vi "Main.vi"() -> ()   [LabVIEW 2021] (continued)
                    n1024 = String Subset(string=w1278, length (rest)=16 ("长度（剩余）")) -> (substring=w1277:string)  [unwired: 1 in]
                    n1025 = property on="曲线49设置" class="Str"("Val(Sgnl)"=w1277) -> ()  [unwired: 2 in, 2 out]
                    n1026 = invoke on="控件配置文件" class="Tbl (严格)" method="Set Cell Value"("X Index"=1 ("X索引"), "Y Index"=w1272, "Value"=w1279) -> ()  [unwired: 3 in, 6 out]
                    n1027 = invoke on="控件配置文件" class="Tbl (严格)" method="Set Cell Value"("X Index"=0 ("X索引"), "Y Index"=w1272, "Value"=w1277) -> ()  [unwired: 3 in, 6 out]
                  }
                  frame "关联到曲线50" {
                    w1283 = T9 79 items=["刷新间隔", "波特率", "布尔1设置项", "布尔2设置项", "布尔3设置项", "布尔4设置项", "布尔5设置项", "布尔6设置项", "布尔7设置项", "布尔8设置项", "显控1设置", "显控2设置", "显控3设置", "显控4设置", "显控5设置", "显控6设置", "显控7设置", "显控8设置", "显控9设置", "显控10设置", "显控11设置", "显控12设置", "设控1设置", "设控2设置", "设控3设置", "设控4设置", "设控5设置", "设控6设置", "设控7设置", "设控8设置", "曲线1设置", "曲线2设置", "曲线3设置", "曲线4设置", "曲线5设置", "曲线6设置", "曲线7设置", "曲线8设置", "曲线9设置", "曲线10设置", "曲线11设置", "曲线12设置", "曲线13设置", "曲线14设置", "曲线15设置", "曲线16设置", "曲线17设置", "曲线18设置", "曲线19设置", "曲线20设置", "曲线21设置", "曲线22设置", "曲线23设置", "曲线24设置", "曲线25设置", "曲线26设置", "曲线27设置", "曲线28设置", "曲线29设置", "曲线30设置", "曲线31设置", "曲线32设置", "曲线33设置", "曲线34设置", "曲线35设置", "曲线36设置", "曲线37设置", "曲线38设置", "曲线39设置", "曲线40设置", "曲线41设置", "曲线42设置", "曲线43设置", "曲线44设置", "曲线45设置", "曲线46设置", "曲线47设置", "曲线48设置", "曲线49设置", "曲线50设置", "曲线51设置", "曲线52设置", "曲线53设置", "曲线54设置", "曲线55设置", "曲线56设置", "曲线57设置", "曲线58设置", "曲线59设置", "曲线60设置", "曲线61设置", "曲线62设置", "曲线63设置", "曲线64设置", "ID值", "数据模式"] ("DataInitDef")
                    n1028 = property on="表格" class="Tbl (严格)"() -> ("Selection Start"=w1293:T1)  [unwired: 2 in, 2 out]
                    n1029 = Unbundle By Name(w1293) -> ("Row"=w1291:i32)
                    n1030 = property on="表格" class="Tbl (严格)"() -> ("Value"=w1292:string[][])  [unwired: 2 in, 2 out]
                    n1031 = Number To Decimal String(number=w1291) -> (decimal integer string=w1290:string)  [unwired: 1 in]
                    n1032 = Index Array(array=w1292, index (row)=w1291, index (col)=0 ("禁用的索引 (列)")) -> (element=w1289:string)
                    n1033 = String Subset(string=w1289, length (rest)=16 ("长度（剩余）")) -> (substring=w1288:string)  [unwired: 1 in]
                    n1034 = property on="曲线50设置" class="Str"("Val(Sgnl)"=w1288) -> ()  [unwired: 2 in, 2 out]
                    n1035 = invoke on="控件配置文件" class="Tbl (严格)" method="Set Cell Value"("X Index"=1 ("X索引"), "Y Index"=w1283, "Value"=w1290) -> ()  [unwired: 3 in, 6 out]
                    n1036 = invoke on="控件配置文件" class="Tbl (严格)" method="Set Cell Value"("X Index"=0 ("X索引"), "Y Index"=w1283, "Value"=w1288) -> ()  [unwired: 3 in, 6 out]
                  }
                  frame "关联到曲线51" {
                    w1294 = T9 80 items=["刷新间隔", "波特率", "布尔1设置项", "布尔2设置项", "布尔3设置项", "布尔4设置项", "布尔5设置项", "布尔6设置项", "布尔7设置项", "布尔8设置项", "显控1设置", "显控2设置", "显控3设置", "显控4设置", "显控5设置", "显控6设置", "显控7设置", "显控8设置", "显控9设置", "显控10设置", "显控11设置", "显控12设置", "设控1设置", "设控2设置", "设控3设置", "设控4设置", "设控5设置", "设控6设置", "设控7设置", "设控8设置", "曲线1设置", "曲线2设置", "曲线3设置", "曲线4设置", "曲线5设置", "曲线6设置", "曲线7设置", "曲线8设置", "曲线9设置", "曲线10设置", "曲线11设置", "曲线12设置", "曲线13设置", "曲线14设置", "曲线15设置", "曲线16设置", "曲线17设置", "曲线18设置", "曲线19设置", "曲线20设置", "曲线21设置", "曲线22设置", "曲线23设置", "曲线24设置", "曲线25设置", "曲线26设置", "曲线27设置", "曲线28设置", "曲线29设置", "曲线30设置", "曲线31设置", "曲线32设置", "曲线33设置", "曲线34设置", "曲线35设置", "曲线36设置", "曲线37设置", "曲线38设置", "曲线39设置", "曲线40设置", "曲线41设置", "曲线42设置", "曲线43设置", "曲线44设置", "曲线45设置", "曲线46设置", "曲线47设置", "曲线48设置", "曲线49设置", "曲线50设置", "曲线51设置", "曲线52设置", "曲线53设置", "曲线54设置", "曲线55设置", "曲线56设置", "曲线57设置", "曲线58设置", "曲线59设置", "曲线60设置", "曲线61设置", "曲线62设置", "曲线63设置", "曲线64设置", "ID值", "数据模式"] ("DataInitDef")
                    n1037 = property on="表格" class="Tbl (严格)"() -> ("Selection Start"=w1304:T1)  [unwired: 2 in, 2 out]
                    n1038 = Unbundle By Name(w1304) -> ("Row"=w1302:i32)
                    n1039 = property on="表格" class="Tbl (严格)"() -> ("Value"=w1303:string[][])  [unwired: 2 in, 2 out]
                    n1040 = Number To Decimal String(number=w1302) -> (decimal integer string=w1301:string)  [unwired: 1 in]
                    n1041 = Index Array(array=w1303, index (row)=w1302, index (col)=0 ("禁用的索引 (列)")) -> (element=w1300:string)
                    n1042 = String Subset(string=w1300, length (rest)=16 ("长度（剩余）")) -> (substring=w1299:string)  [unwired: 1 in]
                    n1043 = property on="曲线51设置" class="Str"("Val(Sgnl)"=w1299) -> ()  [unwired: 2 in, 2 out]
                    n1044 = invoke on="控件配置文件" class="Tbl (严格)" method="Set Cell Value"("X Index"=1 ("X索引"), "Y Index"=w1294, "Value"=w1301) -> ()  [unwired: 3 in, 6 out]
                    n1045 = invoke on="控件配置文件" class="Tbl (严格)" method="Set Cell Value"("X Index"=0 ("X索引"), "Y Index"=w1294, "Value"=w1299) -> ()  [unwired: 3 in, 6 out]
                  }
                  frame "关联到曲线52" {
                    w1305 = T9 81 items=["刷新间隔", "波特率", "布尔1设置项", "布尔2设置项", "布尔3设置项", "布尔4设置项", "布尔5设置项", "布尔6设置项", "布尔7设置项", "布尔8设置项", "显控1设置", "显控2设置", "显控3设置", "显控4设置", "显控5设置", "显控6设置", "显控7设置", "显控8设置", "显控9设置", "显控10设置", "显控11设置", "显控12设置", "设控1设置", "设控2设置", "设控3设置", "设控4设置", "设控5设置", "设控6设置", "设控7设置", "设控8设置", "曲线1设置", "曲线2设置", "曲线3设置", "曲线4设置", "曲线5设置", "曲线6设置", "曲线7设置", "曲线8设置", "曲线9设置", "曲线10设置", "曲线11设置", "曲线12设置", "曲线13设置", "曲线14设置", "曲线15设置", "曲线16设置", "曲线17设置", "曲线18设置", "曲线19设置", "曲线20设置", "曲线21设置", "曲线22设置", "曲线23设置", "曲线24设置", "曲线25设置", "曲线26设置", "曲线27设置", "曲线28设置", "曲线29设置", "曲线30设置", "曲线31设置", "曲线32设置", "曲线33设置", "曲线34设置", "曲线35设置", "曲线36设置", "曲线37设置", "曲线38设置", "曲线39设置", "曲线40设置", "曲线41设置", "曲线42设置", "曲线43设置", "曲线44设置", "曲线45设置", "曲线46设置", "曲线47设置", "曲线48设置", "曲线49设置", "曲线50设置", "曲线51设置", "曲线52设置", "曲线53设置", "曲线54设置", "曲线55设置", "曲线56设置", "曲线57设置", "曲线58设置", "曲线59设置", "曲线60设置", "曲线61设置", "曲线62设置", "曲线63设置", "曲线64设置", "ID值", "数据模式"] ("DataInitDef")
                    n1046 = property on="表格" class="Tbl (严格)"() -> ("Selection Start"=w1315:T1)  [unwired: 2 in, 2 out]
                    n1047 = Unbundle By Name(w1315) -> ("Row"=w1313:i32)
                    n1048 = property on="表格" class="Tbl (严格)"() -> ("Value"=w1314:string[][])  [unwired: 2 in, 2 out]
                    n1049 = Number To Decimal String(number=w1313) -> (decimal integer string=w1312:string)  [unwired: 1 in]
                    n1050 = Index Array(array=w1314, index (row)=w1313, index (col)=0 ("禁用的索引 (列)")) -> (element=w1311:string)
                    n1051 = String Subset(string=w1311, length (rest)=16 ("长度（剩余）")) -> (substring=w1310:string)  [unwired: 1 in]
                    n1052 = property on="曲线52设置" class="Str"("Val(Sgnl)"=w1310) -> ()  [unwired: 2 in, 2 out]
                    n1053 = invoke on="控件配置文件" class="Tbl (严格)" method="Set Cell Value"("X Index"=1 ("X索引"), "Y Index"=w1305, "Value"=w1312) -> ()  [unwired: 3 in, 6 out]
                    n1054 = invoke on="控件配置文件" class="Tbl (严格)" method="Set Cell Value"("X Index"=0 ("X索引"), "Y Index"=w1305, "Value"=w1310) -> ()  [unwired: 3 in, 6 out]
                  }
                  frame "关联到曲线53" {
                    w1316 = T9 82 items=["刷新间隔", "波特率", "布尔1设置项", "布尔2设置项", "布尔3设置项", "布尔4设置项", "布尔5设置项", "布尔6设置项", "布尔7设置项", "布尔8设置项", "显控1设置", "显控2设置", "显控3设置", "显控4设置", "显控5设置", "显控6设置", "显控7设置", "显控8设置", "显控9设置", "显控10设置", "显控11设置", "显控12设置", "设控1设置", "设控2设置", "设控3设置", "设控4设置", "设控5设置", "设控6设置", "设控7设置", "设控8设置", "曲线1设置", "曲线2设置", "曲线3设置", "曲线4设置", "曲线5设置", "曲线6设置", "曲线7设置", "曲线8设置", "曲线9设置", "曲线10设置", "曲线11设置", "曲线12设置", "曲线13设置", "曲线14设置", "曲线15设置", "曲线16设置", "曲线17设置", "曲线18设置", "曲线19设置", "曲线20设置", "曲线21设置", "曲线22设置", "曲线23设置", "曲线24设置", "曲线25设置", "曲线26设置", "曲线27设置", "曲线28设置", "曲线29设置", "曲线30设置", "曲线31设置", "曲线32设置", "曲线33设置", "曲线34设置", "曲线35设置", "曲线36设置", "曲线37设置", "曲线38设置", "曲线39设置", "曲线40设置", "曲线41设置", "曲线42设置", "曲线43设置", "曲线44设置", "曲线45设置", "曲线46设置", "曲线47设置", "曲线48设置", "曲线49设置", "曲线50设置", "曲线51设置", "曲线52设置", "曲线53设置", "曲线54设置", "曲线55设置", "曲线56设置", "曲线57设置", "曲线58设置", "曲线59设置", "曲线60设置", "曲线61设置", "曲线62设置", "曲线63设置", "曲线64设置", "ID值", "数据模式"] ("DataInitDef")
                    n1055 = property on="表格" class="Tbl (严格)"() -> ("Selection Start"=w1326:T1)  [unwired: 2 in, 2 out]
                    n1056 = Unbundle By Name(w1326) -> ("Row"=w1324:i32)
                    n1057 = property on="表格" class="Tbl (严格)"() -> ("Value"=w1325:string[][])  [unwired: 2 in, 2 out]
                    n1058 = Number To Decimal String(number=w1324) -> (decimal integer string=w1323:string)  [unwired: 1 in]
                    n1059 = Index Array(array=w1325, index (row)=w1324, index (col)=0 ("禁用的索引 (列)")) -> (element=w1322:string)
                    n1060 = String Subset(string=w1322, length (rest)=16 ("长度（剩余）")) -> (substring=w1321:string)  [unwired: 1 in]
                    n1061 = property on="曲线53设置" class="Str"("Val(Sgnl)"=w1321) -> ()  [unwired: 2 in, 2 out]
                    n1062 = invoke on="控件配置文件" class="Tbl (严格)" method="Set Cell Value"("X Index"=1 ("X索引"), "Y Index"=w1316, "Value"=w1323) -> ()  [unwired: 3 in, 6 out]
                    n1063 = invoke on="控件配置文件" class="Tbl (严格)" method="Set Cell Value"("X Index"=0 ("X索引"), "Y Index"=w1316, "Value"=w1321) -> ()  [unwired: 3 in, 6 out]
                  }
                  frame "关联到曲线54" {
                    w1327 = T9 83 items=["刷新间隔", "波特率", "布尔1设置项", "布尔2设置项", "布尔3设置项", "布尔4设置项", "布尔5设置项", "布尔6设置项", "布尔7设置项", "布尔8设置项", "显控1设置", "显控2设置", "显控3设置", "显控4设置", "显控5设置", "显控6设置", "显控7设置", "显控8设置", "显控9设置", "显控10设置", "显控11设置", "显控12设置", "设控1设置", "设控2设置", "设控3设置", "设控4设置", "设控5设置", "设控6设置", "设控7设置", "设控8设置", "曲线1设置", "曲线2设置", "曲线3设置", "曲线4设置", "曲线5设置", "曲线6设置", "曲线7设置", "曲线8设置", "曲线9设置", "曲线10设置", "曲线11设置", "曲线12设置", "曲线13设置", "曲线14设置", "曲线15设置", "曲线16设置", "曲线17设置", "曲线18设置", "曲线19设置", "曲线20设置", "曲线21设置", "曲线22设置", "曲线23设置", "曲线24设置", "曲线25设置", "曲线26设置", "曲线27设置", "曲线28设置", "曲线29设置", "曲线30设置", "曲线31设置", "曲线32设置", "曲线33设置", "曲线34设置", "曲线35设置", "曲线36设置", "曲线37设置", "曲线38设置", "曲线39设置", "曲线40设置", "曲线41设置", "曲线42设置", "曲线43设置", "曲线44设置", "曲线45设置", "曲线46设置", "曲线47设置", "曲线48设置", "曲线49设置", "曲线50设置", "曲线51设置", "曲线52设置", "曲线53设置", "曲线54设置", "曲线55设置", "曲线56设置", "曲线57设置", "曲线58设置", "曲线59设置", "曲线60设置", "曲线61设置", "曲线62设置", "曲线63设置", "曲线64设置", "ID值", "数据模式"] ("DataInitDef")
                    n1064 = property on="表格" class="Tbl (严格)"() -> ("Selection Start"=w1337:T1)  [unwired: 2 in, 2 out]
                    n1065 = Unbundle By Name(w1337) -> ("Row"=w1335:i32)
                    n1066 = property on="表格" class="Tbl (严格)"() -> ("Value"=w1336:string[][])  [unwired: 2 in, 2 out]
                    n1067 = Number To Decimal String(number=w1335) -> (decimal integer string=w1334:string)  [unwired: 1 in]
                    n1068 = Index Array(array=w1336, index (row)=w1335, index (col)=0 ("禁用的索引 (列)")) -> (element=w1333:string)
                    n1069 = String Subset(string=w1333, length (rest)=16 ("长度（剩余）")) -> (substring=w1332:string)  [unwired: 1 in]
                    n1070 = property on="曲线54设置" class="Str"("Val(Sgnl)"=w1332) -> ()  [unwired: 2 in, 2 out]
                    n1071 = invoke on="控件配置文件" class="Tbl (严格)" method="Set Cell Value"("X Index"=1 ("X索引"), "Y Index"=w1327, "Value"=w1334) -> ()  [unwired: 3 in, 6 out]
                    n1072 = invoke on="控件配置文件" class="Tbl (严格)" method="Set Cell Value"("X Index"=0 ("X索引"), "Y Index"=w1327, "Value"=w1332) -> ()  [unwired: 3 in, 6 out]
                  }
                  frame "关联到曲线55" {
                    w1338 = T9 84 items=["刷新间隔", "波特率", "布尔1设置项", "布尔2设置项", "布尔3设置项", "布尔4设置项", "布尔5设置项", "布尔6设置项", "布尔7设置项", "布尔8设置项", "显控1设置", "显控2设置", "显控3设置", "显控4设置", "显控5设置", "显控6设置", "显控7设置", "显控8设置", "显控9设置", "显控10设置", "显控11设置", "显控12设置", "设控1设置", "设控2设置", "设控3设置", "设控4设置", "设控5设置", "设控6设置", "设控7设置", "设控8设置", "曲线1设置", "曲线2设置", "曲线3设置", "曲线4设置", "曲线5设置", "曲线6设置", "曲线7设置", "曲线8设置", "曲线9设置", "曲线10设置", "曲线11设置", "曲线12设置", "曲线13设置", "曲线14设置", "曲线15设置", "曲线16设置", "曲线17设置", "曲线18设置", "曲线19设置", "曲线20设置", "曲线21设置", "曲线22设置", "曲线23设置", "曲线24设置", "曲线25设置", "曲线26设置", "曲线27设置", "曲线28设置", "曲线29设置", "曲线30设置", "曲线31设置", "曲线32设置", "曲线33设置", "曲线34设置", "曲线35设置", "曲线36设置", "曲线37设置", "曲线38设置", "曲线39设置", "曲线40设置", "曲线41设置", "曲线42设置", "曲线43设置", "曲线44设置", "曲线45设置", "曲线46设置", "曲线47设置", "曲线48设置", "曲线49设置", "曲线50设置", "曲线51设置", "曲线52设置", "曲线53设置", "曲线54设置", "曲线55设置", "曲线56设置", "曲线57设置", "曲线58设置", "曲线59设置", "曲线60设置", "曲线61设置", "曲线62设置", "曲线63设置", "曲线64设置", "ID值", "数据模式"] ("DataInitDef")
                    n1073 = property on="表格" class="Tbl (严格)"() -> ("Selection Start"=w1348:T1)  [unwired: 2 in, 2 out]
                    n1074 = Unbundle By Name(w1348) -> ("Row"=w1346:i32)
                    n1075 = property on="表格" class="Tbl (严格)"() -> ("Value"=w1347:string[][])  [unwired: 2 in, 2 out]
                    n1076 = Number To Decimal String(number=w1346) -> (decimal integer string=w1345:string)  [unwired: 1 in]
                    n1077 = Index Array(array=w1347, index (row)=w1346, index (col)=0 ("禁用的索引 (列)")) -> (element=w1344:string)
                    n1078 = String Subset(string=w1344, length (rest)=16 ("长度（剩余）")) -> (substring=w1343:string)  [unwired: 1 in]
                    n1079 = property on="曲线55设置" class="Str"("Val(Sgnl)"=w1343) -> ()  [unwired: 2 in, 2 out]
                    n1080 = invoke on="控件配置文件" class="Tbl (严格)" method="Set Cell Value"("X Index"=1 ("X索引"), "Y Index"=w1338, "Value"=w1345) -> ()  [unwired: 3 in, 6 out]
                    n1081 = invoke on="控件配置文件" class="Tbl (严格)" method="Set Cell Value"("X Index"=0 ("X索引"), "Y Index"=w1338, "Value"=w1343) -> ()  [unwired: 3 in, 6 out]
                  }
                  frame "关联到曲线56" {
                    w1349 = T9 85 items=["刷新间隔", "波特率", "布尔1设置项", "布尔2设置项", "布尔3设置项", "布尔4设置项", "布尔5设置项", "布尔6设置项", "布尔7设置项", "布尔8设置项", "显控1设置", "显控2设置", "显控3设置", "显控4设置", "显控5设置", "显控6设置", "显控7设置", "显控8设置", "显控9设置", "显控10设置", "显控11设置", "显控12设置", "设控1设置", "设控2设置", "设控3设置", "设控4设置", "设控5设置", "设控6设置", "设控7设置", "设控8设置", "曲线1设置", "曲线2设置", "曲线3设置", "曲线4设置", "曲线5设置", "曲线6设置", "曲线7设置", "曲线8设置", "曲线9设置", "曲线10设置", "曲线11设置", "曲线12设置", "曲线13设置", "曲线14设置", "曲线15设置", "曲线16设置", "曲线17设置", "曲线18设置", "曲线19设置", "曲线20设置", "曲线21设置", "曲线22设置", "曲线23设置", "曲线24设置", "曲线25设置", "曲线26设置", "曲线27设置", "曲线28设置", "曲线29设置", "曲线30设置", "曲线31设置", "曲线32设置", "曲线33设置", "曲线34设置", "曲线35设置", "曲线36设置", "曲线37设置", "曲线38设置", "曲线39设置", "曲线40设置", "曲线41设置", "曲线42设置", "曲线43设置", "曲线44设置", "曲线45设置", "曲线46设置", "曲线47设置", "曲线48设置", "曲线49设置", "曲线50设置", "曲线51设置", "曲线52设置", "曲线53设置", "曲线54设置", "曲线55设置", "曲线56设置", "曲线57设置", "曲线58设置", "曲线59设置", "曲线60设置", "曲线61设置", "曲线62设置", "曲线63设置", "曲线64设置", "ID值", "数据模式"] ("DataInitDef")
                    n1082 = property on="表格" class="Tbl (严格)"() -> ("Selection Start"=w1359:T1)  [unwired: 2 in, 2 out]
                    n1083 = Unbundle By Name(w1359) -> ("Row"=w1357:i32)
                    n1084 = property on="表格" class="Tbl (严格)"() -> ("Value"=w1358:string[][])  [unwired: 2 in, 2 out]
                    n1085 = Number To Decimal String(number=w1357) -> (decimal integer string=w1356:string)  [unwired: 1 in]
                    n1086 = Index Array(array=w1358, index (row)=w1357, index (col)=0 ("禁用的索引 (列)")) -> (element=w1355:string)
                    n1087 = String Subset(string=w1355, length (rest)=16 ("长度（剩余）")) -> (substring=w1354:string)  [unwired: 1 in]
                    n1088 = property on="曲线56设置" class="Str"("Val(Sgnl)"=w1354) -> ()  [unwired: 2 in, 2 out]
                    n1089 = invoke on="控件配置文件" class="Tbl (严格)" method="Set Cell Value"("X Index"=1 ("X索引"), "Y Index"=w1349, "Value"=w1356) -> ()  [unwired: 3 in, 6 out]
                    n1090 = invoke on="控件配置文件" class="Tbl (严格)" method="Set Cell Value"("X Index"=0 ("X索引"), "Y Index"=w1349, "Value"=w1354) -> ()  [unwired: 3 in, 6 out]
                  }
                  frame "关联到曲线57" {
                    w1360 = T9 86 items=["刷新间隔", "波特率", "布尔1设置项", "布尔2设置项", "布尔3设置项", "布尔4设置项", "布尔5设置项", "布尔6设置项", "布尔7设置项", "布尔8设置项", "显控1设置", "显控2设置", "显控3设置", "显控4设置", "显控5设置", "显控6设置", "显控7设置", "显控8设置", "显控9设置", "显控10设置", "显控11设置", "显控12设置", "设控1设置", "设控2设置", "设控3设置", "设控4设置", "设控5设置", "设控6设置", "设控7设置", "设控8设置", "曲线1设置", "曲线2设置", "曲线3设置", "曲线4设置", "曲线5设置", "曲线6设置", "曲线7设置", "曲线8设置", "曲线9设置", "曲线10设置", "曲线11设置", "曲线12设置", "曲线13设置", "曲线14设置", "曲线15设置", "曲线16设置", "曲线17设置", "曲线18设置", "曲线19设置", "曲线20设置", "曲线21设置", "曲线22设置", "曲线23设置", "曲线24设置", "曲线25设置", "曲线26设置", "曲线27设置", "曲线28设置", "曲线29设置", "曲线30设置", "曲线31设置", "曲线32设置", "曲线33设置", "曲线34设置", "曲线35设置", "曲线36设置", "曲线37设置", "曲线38设置", "曲线39设置", "曲线40设置", "曲线41设置", "曲线42设置", "曲线43设置", "曲线44设置", "曲线45设置", "曲线46设置", "曲线47设置", "曲线48设置", "曲线49设置", "曲线50设置", "曲线51设置", "曲线52设置", "曲线53设置", "曲线54设置", "曲线55设置", "曲线56设置", "曲线57设置", "曲线58设置", "曲线59设置", "曲线60设置", "曲线61设置", "曲线62设置", "曲线63设置", "曲线64设置", "ID值", "数据模式"] ("DataInitDef")
                    n1091 = property on="表格" class="Tbl (严格)"() -> ("Selection Start"=w1370:T1)  [unwired: 2 in, 2 out]
                    n1092 = Unbundle By Name(w1370) -> ("Row"=w1368:i32)
                    n1093 = property on="表格" class="Tbl (严格)"() -> ("Value"=w1369:string[][])  [unwired: 2 in, 2 out]
                    n1094 = Number To Decimal String(number=w1368) -> (decimal integer string=w1367:string)  [unwired: 1 in]
                    n1095 = Index Array(array=w1369, index (row)=w1368, index (col)=0 ("禁用的索引 (列)")) -> (element=w1366:string)
                    n1096 = String Subset(string=w1366, length (rest)=16 ("长度（剩余）")) -> (substring=w1365:string)  [unwired: 1 in]
                    n1097 = property on="曲线57设置" class="Str"("Val(Sgnl)"=w1365) -> ()  [unwired: 2 in, 2 out]
                    n1098 = invoke on="控件配置文件" class="Tbl (严格)" method="Set Cell Value"("X Index"=1 ("X索引"), "Y Index"=w1360, "Value"=w1367) -> ()  [unwired: 3 in, 6 out]
                    n1099 = invoke on="控件配置文件" class="Tbl (严格)" method="Set Cell Value"("X Index"=0 ("X索引"), "Y Index"=w1360, "Value"=w1365) -> ()  [unwired: 3 in, 6 out]
                  }
                  frame "关联到曲线58" {
                    w1371 = T9 87 items=["刷新间隔", "波特率", "布尔1设置项", "布尔2设置项", "布尔3设置项", "布尔4设置项", "布尔5设置项", "布尔6设置项", "布尔7设置项", "布尔8设置项", "显控1设置", "显控2设置", "显控3设置", "显控4设置", "显控5设置", "显控6设置", "显控7设置", "显控8设置", "显控9设置", "显控10设置", "显控11设置", "显控12设置", "设控1设置", "设控2设置", "设控3设置", "设控4设置", "设控5设置", "设控6设置", "设控7设置", "设控8设置", "曲线1设置", "曲线2设置", "曲线3设置", "曲线4设置", "曲线5设置", "曲线6设置", "曲线7设置", "曲线8设置", "曲线9设置", "曲线10设置", "曲线11设置", "曲线12设置", "曲线13设置", "曲线14设置", "曲线15设置", "曲线16设置", "曲线17设置", "曲线18设置", "曲线19设置", "曲线20设置", "曲线21设置", "曲线22设置", "曲线23设置", "曲线24设置", "曲线25设置", "曲线26设置", "曲线27设置", "曲线28设置", "曲线29设置", "曲线30设置", "曲线31设置", "曲线32设置", "曲线33设置", "曲线34设置", "曲线35设置", "曲线36设置", "曲线37设置", "曲线38设置", "曲线39设置", "曲线40设置", "曲线41设置", "曲线42设置", "曲线43设置", "曲线44设置", "曲线45设置", "曲线46设置", "曲线47设置", "曲线48设置", "曲线49设置", "曲线50设置", "曲线51设置", "曲线52设置", "曲线53设置", "曲线54设置", "曲线55设置", "曲线56设置", "曲线57设置", "曲线58设置", "曲线59设置", "曲线60设置", "曲线61设置", "曲线62设置", "曲线63设置", "曲线64设置", "ID值", "数据模式"] ("DataInitDef")
                    n1100 = property on="表格" class="Tbl (严格)"() -> ("Selection Start"=w1381:T1)  [unwired: 2 in, 2 out]
                    n1101 = Unbundle By Name(w1381) -> ("Row"=w1379:i32)
                    n1102 = property on="表格" class="Tbl (严格)"() -> ("Value"=w1380:string[][])  [unwired: 2 in, 2 out]
                    n1103 = Number To Decimal String(number=w1379) -> (decimal integer string=w1378:string)  [unwired: 1 in]
                    n1104 = Index Array(array=w1380, index (row)=w1379, index (col)=0 ("禁用的索引 (列)")) -> (element=w1377:string)
                    n1105 = String Subset(string=w1377, length (rest)=16 ("长度（剩余）")) -> (substring=w1376:string)  [unwired: 1 in]
                    n1106 = property on="曲线58设置" class="Str"("Val(Sgnl)"=w1376) -> ()  [unwired: 2 in, 2 out]
                    n1107 = invoke on="控件配置文件" class="Tbl (严格)" method="Set Cell Value"("X Index"=1 ("X索引"), "Y Index"=w1371, "Value"=w1378) -> ()  [unwired: 3 in, 6 out]
                    n1108 = invoke on="控件配置文件" class="Tbl (严格)" method="Set Cell Value"("X Index"=0 ("X索引"), "Y Index"=w1371, "Value"=w1376) -> ()  [unwired: 3 in, 6 out]
                  }
                  frame "关联到曲线59" {
                    w1382 = T9 88 items=["刷新间隔", "波特率", "布尔1设置项", "布尔2设置项", "布尔3设置项", "布尔4设置项", "布尔5设置项", "布尔6设置项", "布尔7设置项", "布尔8设置项", "显控1设置", "显控2设置", "显控3设置", "显控4设置", "显控5设置", "显控6设置", "显控7设置", "显控8设置", "显控9设置", "显控10设置", "显控11设置", "显控12设置", "设控1设置", "设控2设置", "设控3设置", "设控4设置", "设控5设置", "设控6设置", "设控7设置", "设控8设置", "曲线1设置", "曲线2设置", "曲线3设置", "曲线4设置", "曲线5设置", "曲线6设置", "曲线7设置", "曲线8设置", "曲线9设置", "曲线10设置", "曲线11设置", "曲线12设置", "曲线13设置", "曲线14设置", "曲线15设置", "曲线16设置", "曲线17设置", "曲线18设置", "曲线19设置", "曲线20设置", "曲线21设置", "曲线22设置", "曲线23设置", "曲线24设置", "曲线25设置", "曲线26设置", "曲线27设置", "曲线28设置", "曲线29设置", "曲线30设置", "曲线31设置", "曲线32设置", "曲线33设置", "曲线34设置", "曲线35设置", "曲线36设置", "曲线37设置", "曲线38设置", "曲线39设置", "曲线40设置", "曲线41设置", "曲线42设置", "曲线43设置", "曲线44设置", "曲线45设置", "曲线46设置", "曲线47设置", "曲线48设置", "曲线49设置", "曲线50设置", "曲线51设置", "曲线52设置", "曲线53设置", "曲线54设置", "曲线55设置", "曲线56设置", "曲线57设置", "曲线58设置", "曲线59设置", "曲线60设置", "曲线61设置", "曲线62设置", "曲线63设置", "曲线64设置", "ID值", "数据模式"] ("DataInitDef")
                    n1109 = property on="表格" class="Tbl (严格)"() -> ("Selection Start"=w1392:T1)  [unwired: 2 in, 2 out]
                    n1110 = Unbundle By Name(w1392) -> ("Row"=w1390:i32)
                    n1111 = property on="表格" class="Tbl (严格)"() -> ("Value"=w1391:string[][])  [unwired: 2 in, 2 out]
                    n1112 = Number To Decimal String(number=w1390) -> (decimal integer string=w1389:string)  [unwired: 1 in]
                    n1113 = Index Array(array=w1391, index (row)=w1390, index (col)=0 ("禁用的索引 (列)")) -> (element=w1388:string)
                    n1114 = String Subset(string=w1388, length (rest)=16 ("长度（剩余）")) -> (substring=w1387:string)  [unwired: 1 in]
                    n1115 = property on="曲线59设置" class="Str"("Val(Sgnl)"=w1387) -> ()  [unwired: 2 in, 2 out]
                    n1116 = invoke on="控件配置文件" class="Tbl (严格)" method="Set Cell Value"("X Index"=1 ("X索引"), "Y Index"=w1382, "Value"=w1389) -> ()  [unwired: 3 in, 6 out]
                    n1117 = invoke on="控件配置文件" class="Tbl (严格)" method="Set Cell Value"("X Index"=0 ("X索引"), "Y Index"=w1382, "Value"=w1387) -> ()  [unwired: 3 in, 6 out]
                  }
                  frame "关联到曲线60" {
                    w1393 = T9 89 items=["刷新间隔", "波特率", "布尔1设置项", "布尔2设置项", "布尔3设置项", "布尔4设置项", "布尔5设置项", "布尔6设置项", "布尔7设置项", "布尔8设置项", "显控1设置", "显控2设置", "显控3设置", "显控4设置", "显控5设置", "显控6设置", "显控7设置", "显控8设置", "显控9设置", "显控10设置", "显控11设置", "显控12设置", "设控1设置", "设控2设置", "设控3设置", "设控4设置", "设控5设置", "设控6设置", "设控7设置", "设控8设置", "曲线1设置", "曲线2设置", "曲线3设置", "曲线4设置", "曲线5设置", "曲线6设置", "曲线7设置", "曲线8设置", "曲线9设置", "曲线10设置", "曲线11设置", "曲线12设置", "曲线13设置", "曲线14设置", "曲线15设置", "曲线16设置", "曲线17设置", "曲线18设置", "曲线19设置", "曲线20设置", "曲线21设置", "曲线22设置", "曲线23设置", "曲线24设置", "曲线25设置", "曲线26设置", "曲线27设置", "曲线28设置", "曲线29设置", "曲线30设置", "曲线31设置", "曲线32设置", "曲线33设置", "曲线34设置", "曲线35设置", "曲线36设置", "曲线37设置", "曲线38设置", "曲线39设置", "曲线40设置", "曲线41设置", "曲线42设置", "曲线43设置", "曲线44设置", "曲线45设置", "曲线46设置", "曲线47设置", "曲线48设置", "曲线49设置", "曲线50设置", "曲线51设置", "曲线52设置", "曲线53设置", "曲线54设置", "曲线55设置", "曲线56设置", "曲线57设置", "曲线58设置", "曲线59设置", "曲线60设置", "曲线61设置", "曲线62设置", "曲线63设置", "曲线64设置", "ID值", "数据模式"] ("DataInitDef")
                    n1118 = property on="表格" class="Tbl (严格)"() -> ("Selection Start"=w1403:T1)  [unwired: 2 in, 2 out]
                    n1119 = Unbundle By Name(w1403) -> ("Row"=w1401:i32)
                    n1120 = property on="表格" class="Tbl (严格)"() -> ("Value"=w1402:string[][])  [unwired: 2 in, 2 out]
                    n1121 = Number To Decimal String(number=w1401) -> (decimal integer string=w1400:string)  [unwired: 1 in]
                    n1122 = Index Array(array=w1402, index (row)=w1401, index (col)=0 ("禁用的索引 (列)")) -> (element=w1399:string)
                    n1123 = String Subset(string=w1399, length (rest)=16 ("长度（剩余）")) -> (substring=w1398:string)  [unwired: 1 in]
                    n1124 = property on="曲线60设置" class="Str"("Val(Sgnl)"=w1398) -> ()  [unwired: 2 in, 2 out]
                    n1125 = invoke on="控件配置文件" class="Tbl (严格)" method="Set Cell Value"("X Index"=1 ("X索引"), "Y Index"=w1393, "Value"=w1400) -> ()  [unwired: 3 in, 6 out]
                    n1126 = invoke on="控件配置文件" class="Tbl (严格)" method="Set Cell Value"("X Index"=0 ("X索引"), "Y Index"=w1393, "Value"=w1398) -> ()  [unwired: 3 in, 6 out]
                  }
                  frame "关联到曲线61" {
                    w1404 = T9 90 items=["刷新间隔", "波特率", "布尔1设置项", "布尔2设置项", "布尔3设置项", "布尔4设置项", "布尔5设置项", "布尔6设置项", "布尔7设置项", "布尔8设置项", "显控1设置", "显控2设置", "显控3设置", "显控4设置", "显控5设置", "显控6设置", "显控7设置", "显控8设置", "显控9设置", "显控10设置", "显控11设置", "显控12设置", "设控1设置", "设控2设置", "设控3设置", "设控4设置", "设控5设置", "设控6设置", "设控7设置", "设控8设置", "曲线1设置", "曲线2设置", "曲线3设置", "曲线4设置", "曲线5设置", "曲线6设置", "曲线7设置", "曲线8设置", "曲线9设置", "曲线10设置", "曲线11设置", "曲线12设置", "曲线13设置", "曲线14设置", "曲线15设置", "曲线16设置", "曲线17设置", "曲线18设置", "曲线19设置", "曲线20设置", "曲线21设置", "曲线22设置", "曲线23设置", "曲线24设置", "曲线25设置", "曲线26设置", "曲线27设置", "曲线28设置", "曲线29设置", "曲线30设置", "曲线31设置", "曲线32设置", "曲线33设置", "曲线34设置", "曲线35设置", "曲线36设置", "曲线37设置", "曲线38设置", "曲线39设置", "曲线40设置", "曲线41设置", "曲线42设置", "曲线43设置", "曲线44设置", "曲线45设置", "曲线46设置", "曲线47设置", "曲线48设置", "曲线49设置", "曲线50设置", "曲线51设置", "曲线52设置", "曲线53设置", "曲线54设置", "曲线55设置", "曲线56设置", "曲线57设置", "曲线58设置", "曲线59设置", "曲线60设置", "曲线61设置", "曲线62设置", "曲线63设置", "曲线64设置", "ID值", "数据模式"] ("DataInitDef")
                    n1127 = property on="表格" class="Tbl (严格)"() -> ("Selection Start"=w1414:T1)  [unwired: 2 in, 2 out]
                    n1128 = Unbundle By Name(w1414) -> ("Row"=w1412:i32)
                    n1129 = property on="表格" class="Tbl (严格)"() -> ("Value"=w1413:string[][])  [unwired: 2 in, 2 out]
                    n1130 = Number To Decimal String(number=w1412) -> (decimal integer string=w1411:string)  [unwired: 1 in]
                    n1131 = Index Array(array=w1413, index (row)=w1412, index (col)=0 ("禁用的索引 (列)")) -> (element=w1410:string)
                    n1132 = String Subset(string=w1410, length (rest)=16 ("长度（剩余）")) -> (substring=w1409:string)  [unwired: 1 in]
                    n1133 = property on="曲线61设置" class="Str"("Val(Sgnl)"=w1409) -> ()  [unwired: 2 in, 2 out]
                    n1134 = invoke on="控件配置文件" class="Tbl (严格)" method="Set Cell Value"("X Index"=1 ("X索引"), "Y Index"=w1404, "Value"=w1411) -> ()  [unwired: 3 in, 6 out]
                    n1135 = invoke on="控件配置文件" class="Tbl (严格)" method="Set Cell Value"("X Index"=0 ("X索引"), "Y Index"=w1404, "Value"=w1409) -> ()  [unwired: 3 in, 6 out]
                  }
                  frame "关联到曲线62" {
                    w1415 = T9 91 items=["刷新间隔", "波特率", "布尔1设置项", "布尔2设置项", "布尔3设置项", "布尔4设置项", "布尔5设置项", "布尔6设置项", "布尔7设置项", "布尔8设置项", "显控1设置", "显控2设置", "显控3设置", "显控4设置", "显控5设置", "显控6设置", "显控7设置", "显控8设置", "显控9设置", "显控10设置", "显控11设置", "显控12设置", "设控1设置", "设控2设置", "设控3设置", "设控4设置", "设控5设置", "设控6设置", "设控7设置", "设控8设置", "曲线1设置", "曲线2设置", "曲线3设置", "曲线4设置", "曲线5设置", "曲线6设置", "曲线7设置", "曲线8设置", "曲线9设置", "曲线10设置", "曲线11设置", "曲线12设置", "曲线13设置", "曲线14设置", "曲线15设置", "曲线16设置", "曲线17设置", "曲线18设置", "曲线19设置", "曲线20设置", "曲线21设置", "曲线22设置", "曲线23设置", "曲线24设置", "曲线25设置", "曲线26设置", "曲线27设置", "曲线28设置", "曲线29设置", "曲线30设置", "曲线31设置", "曲线32设置", "曲线33设置", "曲线34设置", "曲线35设置", "曲线36设置", "曲线37设置", "曲线38设置", "曲线39设置", "曲线40设置", "曲线41设置", "曲线42设置", "曲线43设置", "曲线44设置", "曲线45设置", "曲线46设置", "曲线47设置", "曲线48设置", "曲线49设置", "曲线50设置", "曲线51设置", "曲线52设置", "曲线53设置", "曲线54设置", "曲线55设置", "曲线56设置", "曲线57设置", "曲线58设置", "曲线59设置", "曲线60设置", "曲线61设置", "曲线62设置", "曲线63设置", "曲线64设置", "ID值", "数据模式"] ("DataInitDef")
                    n1136 = property on="表格" class="Tbl (严格)"() -> ("Selection Start"=w1425:T1)  [unwired: 2 in, 2 out]
                    n1137 = Unbundle By Name(w1425) -> ("Row"=w1423:i32)
                    n1138 = property on="表格" class="Tbl (严格)"() -> ("Value"=w1424:string[][])  [unwired: 2 in, 2 out]
                    n1139 = Number To Decimal String(number=w1423) -> (decimal integer string=w1422:string)  [unwired: 1 in]
                    n1140 = Index Array(array=w1424, index (row)=w1423, index (col)=0 ("禁用的索引 (列)")) -> (element=w1421:string)
                    n1141 = String Subset(string=w1421, length (rest)=16 ("长度（剩余）")) -> (substring=w1420:string)  [unwired: 1 in]
                    n1142 = property on="曲线62设置" class="Str"("Val(Sgnl)"=w1420) -> ()  [unwired: 2 in, 2 out]
                    n1143 = invoke on="控件配置文件" class="Tbl (严格)" method="Set Cell Value"("X Index"=1 ("X索引"), "Y Index"=w1415, "Value"=w1422) -> ()  [unwired: 3 in, 6 out]
                    n1144 = invoke on="控件配置文件" class="Tbl (严格)" method="Set Cell Value"("X Index"=0 ("X索引"), "Y Index"=w1415, "Value"=w1420) -> ()  [unwired: 3 in, 6 out]
                  }
                  frame "关联到曲线63" {
                    w1426 = T9 92 items=["刷新间隔", "波特率", "布尔1设置项", "布尔2设置项", "布尔3设置项", "布尔4设置项", "布尔5设置项", "布尔6设置项", "布尔7设置项", "布尔8设置项", "显控1设置", "显控2设置", "显控3设置", "显控4设置", "显控5设置", "显控6设置", "显控7设置", "显控8设置", "显控9设置", "显控10设置", "显控11设置", "显控12设置", "设控1设置", "设控2设置", "设控3设置", "设控4设置", "设控5设置", "设控6设置", "设控7设置", "设控8设置", "曲线1设置", "曲线2设置", "曲线3设置", "曲线4设置", "曲线5设置", "曲线6设置", "曲线7设置", "曲线8设置", "曲线9设置", "曲线10设置", "曲线11设置", "曲线12设置", "曲线13设置", "曲线14设置", "曲线15设置", "曲线16设置", "曲线17设置", "曲线18设置", "曲线19设置", "曲线20设置", "曲线21设置", "曲线22设置", "曲线23设置", "曲线24设置", "曲线25设置", "曲线26设置", "曲线27设置", "曲线28设置", "曲线29设置", "曲线30设置", "曲线31设置", "曲线32设置", "曲线33设置", "曲线34设置", "曲线35设置", "曲线36设置", "曲线37设置", "曲线38设置", "曲线39设置", "曲线40设置", "曲线41设置", "曲线42设置", "曲线43设置", "曲线44设置", "曲线45设置", "曲线46设置", "曲线47设置", "曲线48设置", "曲线49设置", "曲线50设置", "曲线51设置", "曲线52设置", "曲线53设置", "曲线54设置", "曲线55设置", "曲线56设置", "曲线57设置", "曲线58设置", "曲线59设置", "曲线60设置", "曲线61设置", "曲线62设置", "曲线63设置", "曲线64设置", "ID值", "数据模式"] ("DataInitDef")
                    n1145 = property on="表格" class="Tbl (严格)"() -> ("Selection Start"=w1436:T1)  [unwired: 2 in, 2 out]
                    n1146 = Unbundle By Name(w1436) -> ("Row"=w1434:i32)
                    n1147 = property on="表格" class="Tbl (严格)"() -> ("Value"=w1435:string[][])  [unwired: 2 in, 2 out]
                    n1148 = Number To Decimal String(number=w1434) -> (decimal integer string=w1433:string)  [unwired: 1 in]
                    n1149 = Index Array(array=w1435, index (row)=w1434, index (col)=0 ("禁用的索引 (列)")) -> (element=w1432:string)
                    n1150 = String Subset(string=w1432, length (rest)=16 ("长度（剩余）")) -> (substring=w1431:string)  [unwired: 1 in]
                    n1151 = property on="曲线63设置" class="Str"("Val(Sgnl)"=w1431) -> ()  [unwired: 2 in, 2 out]
                    n1152 = invoke on="控件配置文件" class="Tbl (严格)" method="Set Cell Value"("X Index"=1 ("X索引"), "Y Index"=w1426, "Value"=w1433) -> ()  [unwired: 3 in, 6 out]
                    n1153 = invoke on="控件配置文件" class="Tbl (严格)" method="Set Cell Value"("X Index"=0 ("X索引"), "Y Index"=w1426, "Value"=w1431) -> ()  [unwired: 3 in, 6 out]
                  }
                  frame "关联到曲线64" {
                    w1437 = T9 93 items=["刷新间隔", "波特率", "布尔1设置项", "布尔2设置项", "布尔3设置项", "布尔4设置项", "布尔5设置项", "布尔6设置项", "布尔7设置项", "布尔8设置项", "显控1设置", "显控2设置", "显控3设置", "显控4设置", "显控5设置", "显控6设置", "显控7设置", "显控8设置", "显控9设置", "显控10设置", "显控11设置", "显控12设置", "设控1设置", "设控2设置", "设控3设置", "设控4设置", "设控5设置", "设控6设置", "设控7设置", "设控8设置", "曲线1设置", "曲线2设置", "曲线3设置", "曲线4设置", "曲线5设置", "曲线6设置", "曲线7设置", "曲线8设置", "曲线9设置", "曲线10设置", "曲线11设置", "曲线12设置", "曲线13设置", "曲线14设置", "曲线15设置", "曲线16设置", "曲线17设置", "曲线18设置", "曲线19设置", "曲线20设置", "曲线21设置", "曲线22设置", "曲线23设置", "曲线24设置", "曲线25设置", "曲线26设置", "曲线27设置", "曲线28设置", "曲线29设置", "曲线30设置", "曲线31设置", "曲线32设置", "曲线33设置", "曲线34设置", "曲线35设置", "曲线36设置", "曲线37设置", "曲线38设置", "曲线39设置", "曲线40设置", "曲线41设置", "曲线42设置", "曲线43设置", "曲线44设置", "曲线45设置", "曲线46设置", "曲线47设置", "曲线48设置", "曲线49设置", "曲线50设置", "曲线51设置", "曲线52设置", "曲线53设置", "曲线54设置", "曲线55设置", "曲线56设置", "曲线57设置", "曲线58设置", "曲线59设置", "曲线60设置", "曲线61设置", "曲线62设置", "曲线63设置", "曲线64设置", "ID值", "数据模式"] ("DataInitDef")
                    n1154 = property on="表格" class="Tbl (严格)"() -> ("Selection Start"=w1447:T1)  [unwired: 2 in, 2 out]
                    n1155 = Unbundle By Name(w1447) -> ("Row"=w1445:i32)
                    n1156 = property on="表格" class="Tbl (严格)"() -> ("Value"=w1446:string[][])  [unwired: 2 in, 2 out]
                    n1157 = Number To Decimal String(number=w1445) -> (decimal integer string=w1444:string)  [unwired: 1 in]
                    n1158 = Index Array(array=w1446, index (row)=w1445, index (col)=0 ("禁用的索引 (列)")) -> (element=w1443:string)
                    n1159 = String Subset(string=w1443, length (rest)=16 ("长度（剩余）")) -> (substring=w1442:string)  [unwired: 1 in]
                    n1160 = property on="曲线64设置" class="Str"("Val(Sgnl)"=w1442) -> ()  [unwired: 2 in, 2 out]
                    n1161 = invoke on="控件配置文件" class="Tbl (严格)" method="Set Cell Value"("X Index"=1 ("X索引"), "Y Index"=w1437, "Value"=w1444) -> ()  [unwired: 3 in, 6 out]
                    n1162 = invoke on="控件配置文件" class="Tbl (严格)" method="Set Cell Value"("X Index"=0 ("X索引"), "Y Index"=w1437, "Value"=w1442) -> ()  [unwired: 3 in, 6 out]
                  }
                  frame "关联到设控1" {
                    w1448 = T9 22 items=["刷新间隔", "波特率", "布尔1设置项", "布尔2设置项", "布尔3设置项", "布尔4设置项", "布尔5设置项", "布尔6设置项", "布尔7设置项", "布尔8设置项", "显控1设置", "显控2设置", "显控3设置", "显控4设置", "显控5设置", "显控6设置", "显控7设置", "显控8设置", "显控9设置", "显控10设置", "显控11设置", "显控12设置", "设控1设置", "设控2设置", "设控3设置", "设控4设置", "设控5设置", "设控6设置", "设控7设置", "设控8设置", "曲线1设置", "曲线2设置", "曲线3设置", "曲线4设置", "曲线5设置", "曲线6设置", "曲线7设置", "曲线8设置", "曲线9设置", "曲线10设置", "曲线11设置", "曲线12设置", "曲线13设置", "曲线14设置", "曲线15设置", "曲线16设置", "曲线17设置", "曲线18设置", "曲线19设置", "曲线20设置", "曲线21设置", "曲线22设置", "曲线23设置", "曲线24设置", "曲线25设置", "曲线26设置", "曲线27设置", "曲线28设置", "曲线29设置", "曲线30设置", "曲线31设置", "曲线32设置", "曲线33设置", "曲线34设置", "曲线35设置", "曲线36设置", "曲线37设置", "曲线38设置", "曲线39设置", "曲线40设置", "曲线41设置", "曲线42设置", "曲线43设置", "曲线44设置", "曲线45设置", "曲线46设置", "曲线47设置", "曲线48设置", "曲线49设置", "曲线50设置", "曲线51设置", "曲线52设置", "曲线53设置", "曲线54设置", "曲线55设置", "曲线56设置", "曲线57设置", "曲线58设置", "曲线59设置", "曲线60设置", "曲线61设置", "曲线62设置", "曲线63设置", "曲线64设置", "ID值", "数据模式"] ("DataInitDef")
                    n1163 = property on="表格" class="Tbl (严格)"() -> ("Selection Start"=w1457:T1)  [unwired: 2 in, 2 out]
                    n1164 = Unbundle By Name(w1457) -> ("Row"=w1455:i32)
                    n1165 = property on="表格" class="Tbl (严格)"() -> ("Value"=w1456:string[][])  [unwired: 2 in, 2 out]
                    n1166 = Number To Decimal String(number=w1455) -> (decimal integer string=w1452:string)  [unwired: 1 in]
                    n1167 = Index Array(array=w1456, index (row)=w1455, index (col)=0 ("禁用的索引 (列)")) -> (element=w1450:string)
                    n1168 = String Subset(string=w1450, length (rest)=16 ("长度（剩余）")) -> (substring=w1449:string)  [unwired: 1 in]
                    n1169 = invoke on="控件配置文件" class="Tbl (严格)" method="Set Cell Value"("X Index"=1 ("X索引"), "Y Index"=w1448, "Value"=w1452) -> ()  [unwired: 3 in, 6 out]
                    n1170 = property on="设控1" class="Str"("Caption.Text"=w1449) -> ()  [unwired: 2 in, 2 out]
                    n1171 = property on="设控设置 1" class="Str"("Val(Sgnl)"=w1449) -> ()  [unwired: 2 in, 2 out]
                    n1172 = invoke on="控件配置文件" class="Tbl (严格)" method="Set Cell Value"("X Index"=0 ("X索引"), "Y Index"=w1448, "Value"=w1449) -> ()  [unwired: 3 in, 6 out]
                  }
                  frame "关联到设控2" {
                    w1459 = T9 23 items=["刷新间隔", "波特率", "布尔1设置项", "布尔2设置项", "布尔3设置项", "布尔4设置项", "布尔5设置项", "布尔6设置项", "布尔7设置项", "布尔8设置项", "显控1设置", "显控2设置", "显控3设置", "显控4设置", "显控5设置", "显控6设置", "显控7设置", "显控8设置", "显控9设置", "显控10设置", "显控11设置", "显控12设置", "设控1设置", "设控2设置", "设控3设置", "设控4设置", "设控5设置", "设控6设置", "设控7设置", "设控8设置", "曲线1设置", "曲线2设置", "曲线3设置", "曲线4设置", "曲线5设置", "曲线6设置", "曲线7设置", "曲线8设置", "曲线9设置", "曲线10设置", "曲线11设置", "曲线12设置", "曲线13设置", "曲线14设置", "曲线15设置", "曲线16设置", "曲线17设置", "曲线18设置", "曲线19设置", "曲线20设置", "曲线21设置", "曲线22设置", "曲线23设置", "曲线24设置", "曲线25设置", "曲线26设置", "曲线27设置", "曲线28设置", "曲线29设置", "曲线30设置", "曲线31设置", "曲线32设置", "曲线33设置", "曲线34设置", "曲线35设置", "曲线36设置", "曲线37设置", "曲线38设置", "曲线39设置", "曲线40设置", "曲线41设置", "曲线42设置", "曲线43设置", "曲线44设置", "曲线45设置", "曲线46设置", "曲线47设置", "曲线48设置", "曲线49设置", "曲线50设置", "曲线51设置", "曲线52设置", "曲线53设置", "曲线54设置", "曲线55设置", "曲线56设置", "曲线57设置", "曲线58设置", "曲线59设置", "曲线60设置", "曲线61设置", "曲线62设置", "曲线63设置", "曲线64设置", "ID值", "数据模式"] ("DataInitDef")
                    n1173 = property on="表格" class="Tbl (严格)"() -> ("Selection Start"=w1466:T1)  [unwired: 2 in, 2 out]
                    n1174 = Unbundle By Name(w1466) -> ("Row"=w1468:i32)
                    n1175 = property on="表格" class="Tbl (严格)"() -> ("Value"=w1467:string[][])  [unwired: 2 in, 2 out]
                    n1176 = Number To Decimal String(number=w1468) -> (decimal integer string=w1469:string)  [unwired: 1 in]
                    n1177 = Index Array(array=w1467, index (row)=w1468, index (col)=0 ("禁用的索引 (列)")) -> (element=w1461:string)
                    n1178 = String Subset(string=w1461, length (rest)=16 ("长度（剩余）")) -> (substring=w1460:string)  [unwired: 1 in]
                    n1179 = invoke on="控件配置文件" class="Tbl (严格)" method="Set Cell Value"("X Index"=1 ("X索引"), "Y Index"=w1459, "Value"=w1469) -> ()  [unwired: 3 in, 6 out]
                    n1180 = property on="设控2" class="Str"("Caption.Text"=w1460) -> ()  [unwired: 2 in, 2 out]
                    n1181 = property on="设控设置 2" class="Str"("Val(Sgnl)"=w1460) -> ()  [unwired: 2 in, 2 out]
                    n1182 = invoke on="控件配置文件" class="Tbl (严格)" method="Set Cell Value"("X Index"=0 ("X索引"), "Y Index"=w1459, "Value"=w1460) -> ()  [unwired: 3 in, 6 out]
                  }
                  frame "关联到设控3" {
                    w1470 = T9 24 items=["刷新间隔", "波特率", "布尔1设置项", "布尔2设置项", "布尔3设置项", "布尔4设置项", "布尔5设置项", "布尔6设置项", "布尔7设置项", "布尔8设置项", "显控1设置", "显控2设置", "显控3设置", "显控4设置", "显控5设置", "显控6设置", "显控7设置", "显控8设置", "显控9设置", "显控10设置", "显控11设置", "显控12设置", "设控1设置", "设控2设置", "设控3设置", "设控4设置", "设控5设置", "设控6设置", "设控7设置", "设控8设置", "曲线1设置", "曲线2设置", "曲线3设置", "曲线4设置", "曲线5设置", "曲线6设置", "曲线7设置", "曲线8设置", "曲线9设置", "曲线10设置", "曲线11设置", "曲线12设置", "曲线13设置", "曲线14设置", "曲线15设置", "曲线16设置", "曲线17设置", "曲线18设置", "曲线19设置", "曲线20设置", "曲线21设置", "曲线22设置", "曲线23设置", "曲线24设置", "曲线25设置", "曲线26设置", "曲线27设置", "曲线28设置", "曲线29设置", "曲线30设置", "曲线31设置", "曲线32设置", "曲线33设置", "曲线34设置", "曲线35设置", "曲线36设置", "曲线37设置", "曲线38设置", "曲线39设置", "曲线40设置", "曲线41设置", "曲线42设置", "曲线43设置", "曲线44设置", "曲线45设置", "曲线46设置", "曲线47设置", "曲线48设置", "曲线49设置", "曲线50设置", "曲线51设置", "曲线52设置", "曲线53设置", "曲线54设置", "曲线55设置", "曲线56设置", "曲线57设置", "曲线58设置", "曲线59设置", "曲线60设置", "曲线61设置", "曲线62设置", "曲线63设置", "曲线64设置", "ID值", "数据模式"] ("DataInitDef")
                    n1183 = property on="表格" class="Tbl (严格)"() -> ("Selection Start"=w1477:T1)  [unwired: 2 in, 2 out]
                    n1184 = Unbundle By Name(w1477) -> ("Row"=w1479:i32)
                    n1185 = property on="表格" class="Tbl (严格)"() -> ("Value"=w1478:string[][])  [unwired: 2 in, 2 out]
                    n1186 = Number To Decimal String(number=w1479) -> (decimal integer string=w1480:string)  [unwired: 1 in]
                    n1187 = Index Array(array=w1478, index (row)=w1479, index (col)=0 ("禁用的索引 (列)")) -> (element=w1472:string)
                    n1188 = String Subset(string=w1472, length (rest)=16 ("长度（剩余）")) -> (substring=w1471:string)  [unwired: 1 in]
                    n1189 = invoke on="控件配置文件" class="Tbl (严格)" method="Set Cell Value"("X Index"=1 ("X索引"), "Y Index"=w1470, "Value"=w1480) -> ()  [unwired: 3 in, 6 out]
                    n1190 = property on="设控3" class="Str"("Caption.Text"=w1471) -> ()  [unwired: 2 in, 2 out]
                    n1191 = property on="设控设置 3" class="Str"("Val(Sgnl)"=w1471) -> ()  [unwired: 2 in, 2 out]
                    n1192 = invoke on="控件配置文件" class="Tbl (严格)" method="Set Cell Value"("X Index"=0 ("X索引"), "Y Index"=w1470, "Value"=w1471) -> ()  [unwired: 3 in, 6 out]
                  }
                  frame "关联到设控4" {
                    w1481 = T9 25 items=["刷新间隔", "波特率", "布尔1设置项", "布尔2设置项", "布尔3设置项", "布尔4设置项", "布尔5设置项", "布尔6设置项", "布尔7设置项", "布尔8设置项", "显控1设置", "显控2设置", "显控3设置", "显控4设置", "显控5设置", "显控6设置", "显控7设置", "显控8设置", "显控9设置", "显控10设置", "显控11设置", "显控12设置", "设控1设置", "设控2设置", "设控3设置", "设控4设置", "设控5设置", "设控6设置", "设控7设置", "设控8设置", "曲线1设置", "曲线2设置", "曲线3设置", "曲线4设置", "曲线5设置", "曲线6设置", "曲线7设置", "曲线8设置", "曲线9设置", "曲线10设置", "曲线11设置", "曲线12设置", "曲线13设置", "曲线14设置", "曲线15设置", "曲线16设置", "曲线17设置", "曲线18设置", "曲线19设置", "曲线20设置", "曲线21设置", "曲线22设置", "曲线23设置", "曲线24设置", "曲线25设置", "曲线26设置", "曲线27设置", "曲线28设置", "曲线29设置", "曲线30设置", "曲线31设置", "曲线32设置", "曲线33设置", "曲线34设置", "曲线35设置", "曲线36设置", "曲线37设置", "曲线38设置", "曲线39设置", "曲线40设置", "曲线41设置", "曲线42设置", "曲线43设置", "曲线44设置", "曲线45设置", "曲线46设置", "曲线47设置", "曲线48设置", "曲线49设置", "曲线50设置", "曲线51设置", "曲线52设置", "曲线53设置", "曲线54设置", "曲线55设置", "曲线56设置", "曲线57设置", "曲线58设置", "曲线59设置", "曲线60设置", "曲线61设置", "曲线62设置", "曲线63设置", "曲线64设置", "ID值", "数据模式"] ("DataInitDef")
                    n1193 = property on="表格" class="Tbl (严格)"() -> ("Selection Start"=w1491:T1)  [unwired: 2 in, 2 out]
                    n1194 = Unbundle By Name(w1491) -> ("Row"=w1489:i32)
                    n1195 = property on="表格" class="Tbl (严格)"() -> ("Value"=w1490:string[][])  [unwired: 2 in, 2 out]
                    n1196 = Number To Decimal String(number=w1489) -> (decimal integer string=w1488:string)  [unwired: 1 in]
                    n1197 = Index Array(array=w1490, index (row)=w1489, index (col)=0 ("禁用的索引 (列)")) -> (element=w1483:string)
                    n1198 = String Subset(string=w1483, length (rest)=16 ("长度（剩余）")) -> (substring=w1482:string)  [unwired: 1 in]
                    n1199 = invoke on="控件配置文件" class="Tbl (严格)" method="Set Cell Value"("X Index"=1 ("X索引"), "Y Index"=w1481, "Value"=w1488) -> ()  [unwired: 3 in, 6 out]
                    n1200 = property on="设控4" class="Str"("Caption.Text"=w1482) -> ()  [unwired: 2 in, 2 out]
                    n1201 = property on="设控设置 4" class="Str"("Val(Sgnl)"=w1482) -> ()  [unwired: 2 in, 2 out]
                    n1202 = invoke on="控件配置文件" class="Tbl (严格)" method="Set Cell Value"("X Index"=0 ("X索引"), "Y Index"=w1481, "Value"=w1482) -> ()  [unwired: 3 in, 6 out]
                  }
                  frame "关联到设控5" {
                    w1492 = T9 26 items=["刷新间隔", "波特率", "布尔1设置项", "布尔2设置项", "布尔3设置项", "布尔4设置项", "布尔5设置项", "布尔6设置项", "布尔7设置项", "布尔8设置项", "显控1设置", "显控2设置", "显控3设置", "显控4设置", "显控5设置", "显控6设置", "显控7设置", "显控8设置", "显控9设置", "显控10设置", "显控11设置", "显控12设置", "设控1设置", "设控2设置", "设控3设置", "设控4设置", "设控5设置", "设控6设置", "设控7设置", "设控8设置", "曲线1设置", "曲线2设置", "曲线3设置", "曲线4设置", "曲线5设置", "曲线6设置", "曲线7设置", "曲线8设置", "曲线9设置", "曲线10设置", "曲线11设置", "曲线12设置", "曲线13设置", "曲线14设置", "曲线15设置", "曲线16设置", "曲线17设置", "曲线18设置", "曲线19设置", "曲线20设置", "曲线21设置", "曲线22设置", "曲线23设置", "曲线24设置", "曲线25设置", "曲线26设置", "曲线27设置", "曲线28设置", "曲线29设置", "曲线30设置", "曲线31设置", "曲线32设置", "曲线33设置", "曲线34设置", "曲线35设置", "曲线36设置", "曲线37设置", "曲线38设置", "曲线39设置", "曲线40设置", "曲线41设置", "曲线42设置", "曲线43设置", "曲线44设置", "曲线45设置", "曲线46设置", "曲线47设置", "曲线48设置", "曲线49设置", "曲线50设置", "曲线51设置", "曲线52设置", "曲线53设置", "曲线54设置", "曲线55设置", "曲线56设置", "曲线57设置", "曲线58设置", "曲线59设置", "曲线60设置", "曲线61设置", "曲线62设置", "曲线63设置", "曲线64设置", "ID值", "数据模式"] ("DataInitDef")
                    n1203 = property on="表格" class="Tbl (严格)"() -> ("Selection Start"=w1502:T1)  [unwired: 2 in, 2 out]
                    n1204 = Unbundle By Name(w1502) -> ("Row"=w1500:i32)
                    n1205 = property on="表格" class="Tbl (严格)"() -> ("Value"=w1501:string[][])  [unwired: 2 in, 2 out]
                    n1206 = Number To Decimal String(number=w1500) -> (decimal integer string=w1499:string)  [unwired: 1 in]
                    n1207 = Index Array(array=w1501, index (row)=w1500, index (col)=0 ("禁用的索引 (列)")) -> (element=w1494:string)
                    n1208 = String Subset(string=w1494, length (rest)=16 ("长度（剩余）")) -> (substring=w1493:string)  [unwired: 1 in]
                    n1209 = invoke on="控件配置文件" class="Tbl (严格)" method="Set Cell Value"("X Index"=1 ("X索引"), "Y Index"=w1492, "Value"=w1499) -> ()  [unwired: 3 in, 6 out]
                    n1210 = property on="设控5" class="Str"("Caption.Text"=w1493) -> ()  [unwired: 2 in, 2 out]
                    n1211 = property on="设控设置 5" class="Str"("Val(Sgnl)"=w1493) -> ()  [unwired: 2 in, 2 out]
                    n1212 = invoke on="控件配置文件" class="Tbl (严格)" method="Set Cell Value"("X Index"=0 ("X索引"), "Y Index"=w1492, "Value"=w1493) -> ()  [unwired: 3 in, 6 out]
                  }
                  frame "关联到设控6" {
